vi "Count Attendance Result.vi"(6 "ExcuseNotes(\"\")":string[][](array[string]), 8 "error in (no error)":errorcluster, 9 "TimeTables(\"\")":string[][](array[string]), 10 "Calendances(\"\")":string[][](array[string]), 11 "AttendRecord.lvclass":refnum<class "AttendRecord.lvclass">) -> (0 "error out":errorcluster, 3 "AttendRecord.lvclass Out":refnum<class "AttendRecord.lvclass">)   [LabVIEW 2015, in "Admin_Actor.lvlib" / "AttendRecord.lvclass"]
uses:
  AttendRecord.lvclass
  CalAttendance/Type Definitions/NumOfAttendace.ctl
  AttendRecord.lvclass/AttendRecord.ctl
  Setting/g_setting.vi
  Admin_Actor.lvlib
  CalAttendance/CalAttendance.lvclass
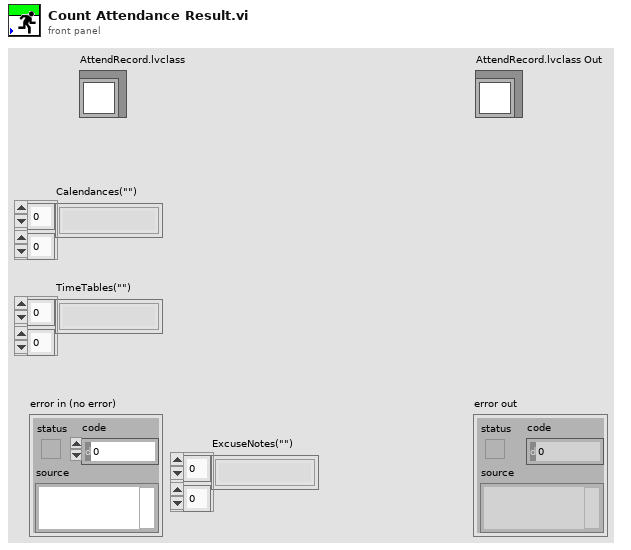
[diagram p1: front panel]
types:
  T1 = typedef "Admin_Actor.lvlib/CalAttendance.lvclass/NumOfAttendace.ctl" = cluster{"TmeOfLate":i32, "TimeOfEarly":i32, "TimeOfExcuse":i32, "TimeOfUnsigned":i32}
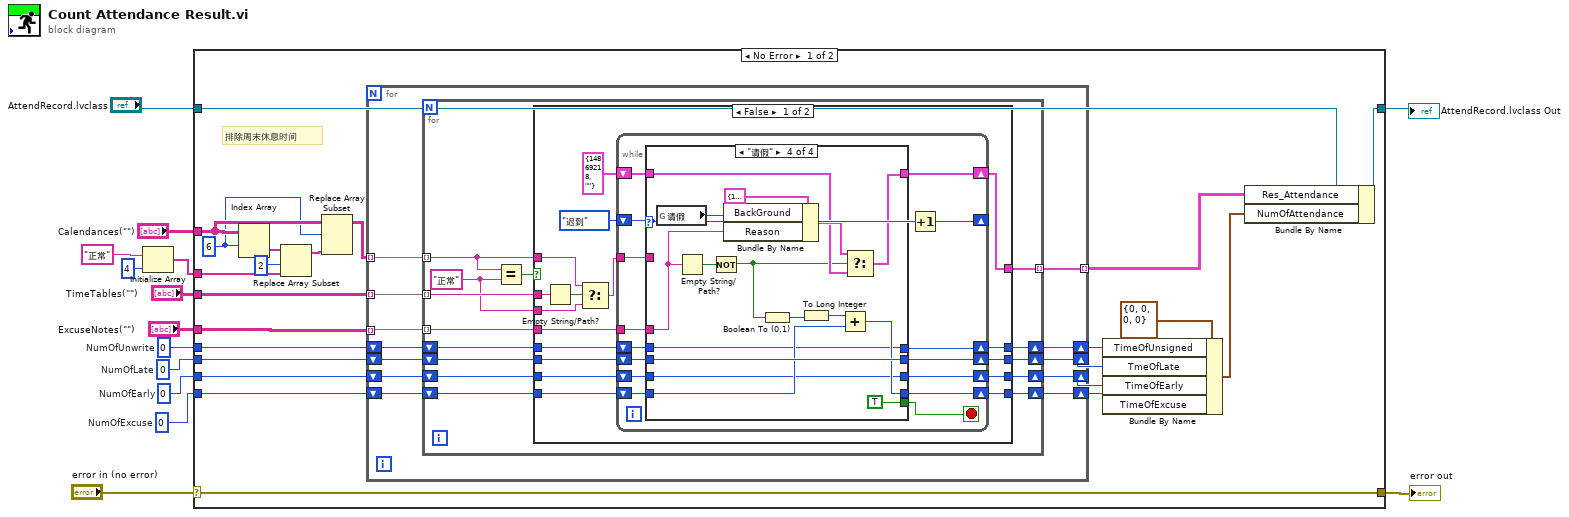
[diagram p0: block diagram]
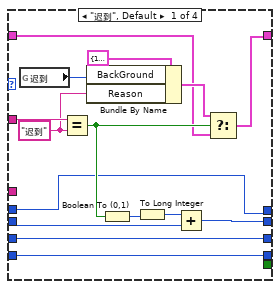
[diagram p2: hidden frame]
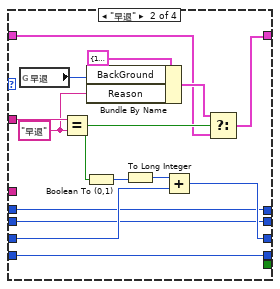
[diagram p3: hidden frame]
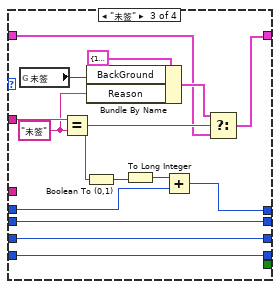
[diagram p4: hidden frame]
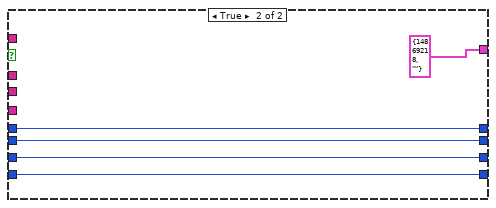
[diagram p5: hidden frame]
diagram:
  w4 = 0  # NumOfUnwrite
  w7 = 0  # NumOfExcuse
  w8 = 0  # NumOfEarly
  w9 = 0  # NumOfLate
  n1 = Initialize Array("正常", 4 ("dimension size")) -> (w1:string[])
  n2 = case shown="No Error" "error in (no error)" {
    selector: "error in (no error)" -> [w37 w163]
    tunnel: [w37 w163] -> w13
    tunnel: [w30 w162] -> w5
    tunnel: "AttendRecord.lvclass" -> [w31 w162]
    tunnel: "Calendances(\"\")" -> [w18 _]
    tunnel: "TimeTables(\"\")" -> [w36 _]
    tunnel: "ExcuseNotes(\"\")" -> [w35 _]
    tunnel: w9 -> [w34 _]
    tunnel: w8 -> [w33 _]
    tunnel: w7 -> [w32 _]
    tunnel: w4 -> [w29 _]
    tunnel: w1 -> [w19 _]
    frame No Error {
      w17 = 6 ("index (row)")
      # "排除周末休息时间"
      n3 = Index Array(array=w18, index (row)=w17) -> (element=w21:string[])  [unwired: 1 in]
      n4 = Replace Array Subset(array=w21, new element=w19, index=2) -> (w16:string[])
      n5 = Replace Array Subset(array=w18, new element=w16, index (row)=w17) -> (w15:string[][])  [unwired: 1 in]
      n6 = for {
        tunnel: w15 -> [w49] mode=indexing
        tunnel: w36 -> [w48] mode=indexing
        tunnel: w35 -> [w47] mode=indexing
        tunnel: [w46] -> w22 mode=indexing
        shift-right: [w42] -> w26
        shift-left: w34 -> [w45]
        shift-right: [w41] -> w25
        shift-left: w33 -> [w44]
        shift-right: [w40] -> w24
        shift-left: w32 -> [w43]
        shift-right: [w38] -> w27
        shift-left: w29 -> [w39]
        n7 = for {
          tunnel: w49 -> [w59] mode=indexing
          tunnel: w48 -> [w61] mode=indexing
          tunnel: w47 -> [w60] mode=indexing
          tunnel: [w62] -> w46 mode=indexing
          shift-right: [w54] -> w42
          shift-left: w45 -> [w57]
          shift-right: [w53] -> w41
          shift-left: w44 -> [w56]
          shift-right: [w52] -> w40
          shift-left: w43 -> [w55]
          shift-right: [w50] -> w38
          shift-left: w39 -> [w51]
          w58 = "正常" ("y")
          n8 = Equal?(x=w59, y=w58) -> (x = y?=w63:bool)
          n9 = case shown="False" w63 {
            tunnel: [w74 cluster{"BackGround":u32, "Reason":string} {"BackGround"=14869218, "Reason"=""} ("Display")] -> w62
            tunnel: w61 -> [w73 _]
            tunnel: w60 -> [w75 _]
            tunnel: w59 -> [w71 _]
            tunnel: w58 -> [w66 _]
            tunnel: w57 -> [w79 w160]
            tunnel: w56 -> [w78 w159]
            tunnel: w55 -> [w77 w158]
            tunnel: [w69 w160] -> w54
            tunnel: [w68 w159] -> w53
            tunnel: [w67 w158] -> w52
            tunnel: w51 -> [w65 w157]
            tunnel: [w64 w157] -> w50
            frame False {
              n10 = Empty String/Path?(string/path=w73) -> (empty?=w72:bool)
              n11 = Select(t=w71, s=w72, f=w66) -> (s? t:f=w70:string)
              n12 = while {
                tunnel: w70 -> [w95]
                shift-right: [w94] -> w74
                shift-left: cluster{"BackGround":u32, "Reason":string} {"BackGround"=14869218, "Reason"=""} ("Display") -> [w93]
                shift-right: [w91] -> _
                shift-left: enum16{"迟到", "早退", "未签", "请假"}."迟到" -> [w92]
                shift-right: [w87] -> w69
                shift-left: w79 -> [w90]
                shift-right: [w86] -> w68
                shift-left: w78 -> [w89]
                shift-right: [w85] -> w67
                shift-left: w77 -> [w88]
                tunnel: w75 -> [w84]
                shift-right: [w81] -> w64
                shift-left: w65 -> [w82]
                stop <- w83 stop-if-true
                n13 = case shown="\"请假\"" w92 {
                  tunnel: w95 -> [w110 w125 w140 _]
                  tunnel: [w105 w120 w135 w153] -> w94
                  tunnel: w93 -> [w99 w116 w131 w150]
                  tunnel: w90 -> [w103 w113 w130 w149]
                  tunnel: w89 -> [w98 w115 w126 w143]
                  tunnel: w88 -> [w97 w112 w129 w145]
                  tunnel: [w100 w113 w130 w149] -> w87
                  tunnel: [w98 w114 w126 w143] -> w86
                  tunnel: [w97 w112 w129 w144] -> w85
                  tunnel: w84 -> [_ _ _ w148]
                  tunnel: [_ _ _ TRUE] -> w83
                  tunnel: w82 -> [w96 w111 w128 w141]
                  tunnel: [w96 w111 w127 w141] -> w81
                  frame "迟到", Default {
                    w107 = "迟到" ("y")
                    n14 = global read "g_setting.vi" "迟到"() -> (w108:u32)
                    n15 = Equal?(x=w110, y=w107) -> (x = y?=w104:bool)
                    n16 = Bundle By Name(cluster=cluster{"BackGround":u32, "Reason":string} {"BackGround"=14869218, "Reason"=""} ("Display"), "BackGround"=w108, "Reason"=w107) -> (w106:cluster{"BackGround":u32, "Reason":string})
                    n17 = Boolean To (0,1)(Boolean=w104) -> (0, 1=w102:i16)
                    n18 = To Long Integer(number=w102) -> (32bit integer=w101:i32)
                    n19 = Add(x=w101, y=w103) -> (x+y=w100:i32)
                    n20 = Select(t=w106, s=w104, f=w99) -> (s? t:f=w105:cluster{"BackGround":u32, "Reason":string})
                  }
                  frame "早退" {
                    w122 = "早退" ("y")
                    n21 = global read "g_setting.vi" "早退"() -> (w123:u32)
                    n22 = Equal?(x=w125, y=w122) -> (x = y?=w119:bool)
                    n23 = Boolean To (0,1)(Boolean=w119) -> (0, 1=w118:i16)
                    n24 = Bundle By Name(cluster=cluster{"BackGround":u32, "Reason":string} {"BackGround"=14869218, "Reason"=""} ("Display"), "BackGround"=w123, "Reason"=w122) -> (w121:cluster{"BackGround":u32, "Reason":string})
                    n25 = To Long Integer(number=w118) -> (32bit integer=w117:i32)
                    n26 = Add(x=w117, y=w115) -> (x+y=w114:i32)
                    n27 = Select(t=w121, s=w119, f=w116) -> (s? t:f=w120:cluster{"BackGround":u32, "Reason":string})
                  }
                  frame "未签" {
                    w137 = "未签" ("y")
                    n28 = global read "g_setting.vi" "未签"() -> (w138:u32)
                    n29 = Equal?(x=w140, y=w137) -> (x = y?=w134:bool)
                    n30 = Boolean To (0,1)(Boolean=w134) -> (0, 1=w133:i16)
                    n31 = Bundle By Name(cluster=cluster{"BackGround":u32, "Reason":string} {"BackGround"=14869218, "Reason"=""} ("Display"), "BackGround"=w138, "Reason"=w137) -> (w136:cluster{"BackGround":u32, "Reason":string})
                    n32 = To Long Integer(number=w133) -> (32bit integer=w132:i32)
                    n33 = Add(x=w132, y=w128) -> (x+y=w127:i32)
                    n34 = Select(t=w136, s=w134, f=w131) -> (s? t:f=w135:cluster{"BackGround":u32, "Reason":string})
                  }
                  frame "请假" {
                    n35 = global read "g_setting.vi" "请假"() -> (w155:u32)
                    n36 = Empty String/Path?(string/path=w148) -> (empty?=w147:bool)
                    n37 = Not(x=w147) -> (.not. x?=w146:bool)
                    n38 = Bundle By Name(cluster=cluster{"BackGround":u32, "Reason":string} {"BackGround"=14869218, "Reason"=""} ("Display"), "BackGround"=w155, "Reason"=w148) -> (w154:cluster{"BackGround":u32, "Reason":string})
                    n39 = Boolean To (0,1)(Boolean=w146) -> (0, 1=w152:i16)
                    n40 = To Long Integer(number=w152) -> (32bit integer=w151:i32)
                    n41 = Add(x=w151, y=w145) -> (x+y=w144:i32)
                    n42 = Select(t=w154, s=w146, f=w150) -> (s? t:f=w153:cluster{"BackGround":u32, "Reason":string})
                  }
                }
                n43 = Increment(x=w92) -> (x+1=w91:enum16{"迟到", "早退", "未签", "请假"})
              }
            }
            frame True {
            }
          }
        }
      }
      n44 = Bundle By Name(cluster=T1 {"TmeOfLate"=0, "TimeOfEarly"=0, "TimeOfExcuse"=0, "TimeOfUnsigned"=0} ("NumOfAttendance"), "TimeOfUnsigned"=w27, "TmeOfLate"=w26, "TimeOfEarly"=w25, "TimeOfExcuse"=w24) -> (w23:T1)
      n45 = Bundle By Name(cluster=w31, "Res_Attendance"=w22, "NumOfAttendance"=w23) -> (w30:refnum<class "AttendRecord.lvclass">)
    }
    frame Error {
    }
  }
  "error out" <- w13
  "AttendRecord.lvclass Out" <- w5
